vi "WL_Joystick Initialization VI.vi"(8 "error in (no error)":errorcluster, 10 "Custom XML":string, 11 "Device Item Ref in":T1 format="%.0x") -> (0 "error out":errorcluster, 3 "Device Item Ref out":T1 format="%.0x")   [LabVIEW 2014, in "WL_Joystick Custom Device.lvlib"]
uses:
  WL_Joystick Custom Device.lvlib
  <vilib>/NI Veristand/Custom Device API/Custom Device Item Ref.ctl
  <vilib>/NI Veristand/Custom Device API/Custom Device Channel.ctl
  <vilib>/NI Veristand/Custom Device API/Custom Device Channel Type.ctl
  <vilib>/NI Veristand/Custom Device API/Custom Device API.lvlib
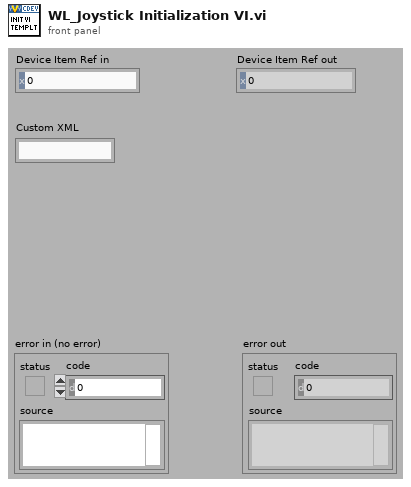
[diagram p1: front panel]
types:
  T1 = typedef "Custom Device API.lvlib/Custom Device Item Ref.ctl" = u64
  T2 = typedef "Custom Device API.lvlib/Custom Device Channel.ctl" = cluster{"Type":T3, "Units":string, "Default Value":dbl, "Faultable":bool, "Scalable":bool}
  T3 = typedef "Custom Device API.lvlib/Custom Device Channel Type.ctl" = enum16{"Input", "Output"}
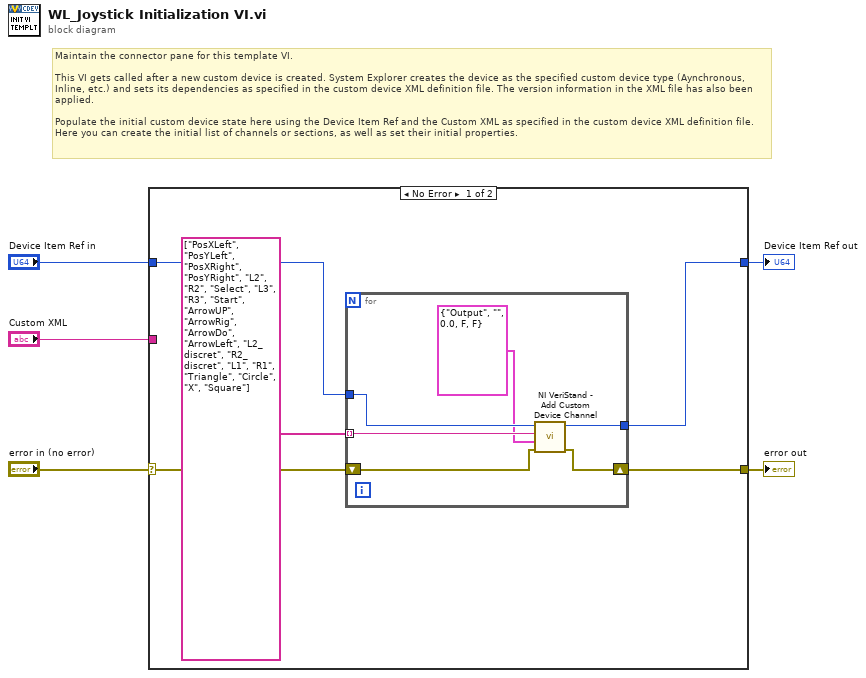
[diagram p0: block diagram]
diagram:
  # "Maintain the connector pane for this template VI.\n\nThis VI gets called after a new custom device is created. System Explorer creates the device as the specified custom device type (Aynchronous, Inline, etc.) and sets its dependencies as specified in the custom device XML definition file. The version information in the XML file has also been applied.\n\nPopulate the initial custom device state here using the Device Item Ref and the Custom XML as specified in the custom device XML definition file. Here you can create the initial list of channels or sections, as well as set their initial properties."
  n1 = case shown="No Error" "error in (no error)" {
    selector: "error in (no error)" -> [w7 w18]
    tunnel: [w6 w18] -> w5
    tunnel: [w8 w17] -> w3
    tunnel: "Device Item Ref in" -> [w9 w17]
    tunnel: "Custom XML" -> [_ _]
    frame No Error {
      n2 = for {
        tunnel: w9 -> [w16]
        tunnel: string[] ["PosXLeft", "PosYLeft", "PosXRight", "PosYRight", "L2", "R2", "Select", "L3", "R3", "Start", "ArrowUP", "ArrowRig", "ArrowDo", "ArrowLeft", "L2_discret", "R2_discret", "L1", "R1", "Triangle", "Circle", "X", "Square"] -> [w15] mode=indexing
        shift-right: [w12] -> w6
        shift-left: w7 -> [w13]
        tunnel: [w11] -> w8
        n3 = call <vilib>:"NI VeriStand - Add Custom Device Channel.vi"("error in (no error)"=w13, "Channel"=T2 {"Type"=enum."Output", "Units"="", "Default Value"=0.0, "Faultable"=FALSE, "Scalable"=FALSE}, "Channel Name"=w15, "Parent Ref in"=w16) -> ("error out"=w12:errorcluster, "Parent Ref out"=w11:T1)  [unwired: 4 in, 2 out]
      }
    }
    frame Error {
    }
  }
  "error out" <- w5
  "Device Item Ref out" <- w3
